vi "Wait For Command.vi"(8 "error in (no error)":errorcluster, 9 "timeout in ms (0)":i32, 11 "Interface in":refnum<class "Interface.lvclass">) -> (0 "error out":errorcluster, 1 "timed out?":bool, 2 "command":T1, 3 "Interface out":refnum<class "Interface.lvclass">, 4 "# elements":u32)   [LabVIEW 2017, in "DSF Core.lvlib" / "Interface.lvclass"]
uses:
  Interface.lvclass
  RT FIFO Data.ctl
  RT FIFO Parameters.ctl
  Interface.lvclass/Interface.ctl
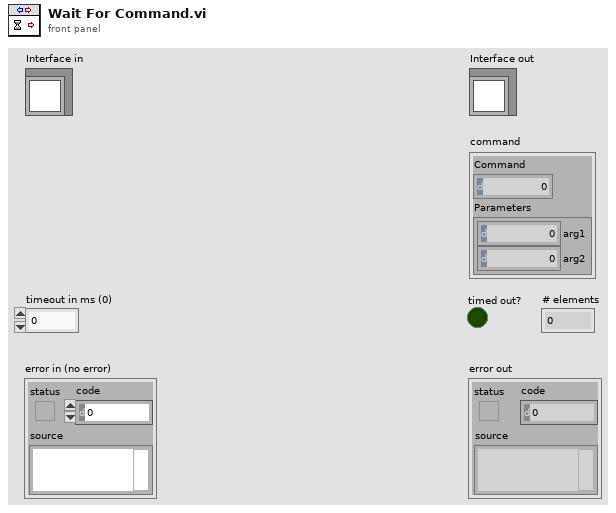
[diagram p1: front panel]
types:
  T1 = typedef "DSF Core.lvlib/Interface.lvclass/RT FIFO Data.ctl" = cluster{"Command":u8, "Parameters":T2}
  T2 = typedef "DSF Core.lvlib/Interface.lvclass/RT FIFO Parameters.ctl" = cluster{"arg1":u64, "arg2":u64}
  T3 = typedef "DSF Core.lvlib/DSF FIFO Options.ctl" = cluster{"Infinite Timeouts":bool}
  T4 = typedef "DSF Core.lvlib/Interface.lvclass/RT FIFO Ref.ctl" = refnum<k33>
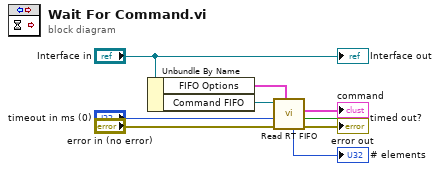
[diagram p0: block diagram]
diagram:
  n1 = Unbundle By Name("Interface in") -> ("FIFO Options"=w1:T3, "Command FIFO"=w2:T4)
  n2 = call "Read RT FIFO.vi"("FIFO Options"=w1, "error in (no error)"="error in (no error)", "timeout in ms (0)"="timeout in ms (0)", "RT FIFO in"=w2) -> ("error out"=→"error out":errorcluster, "empty?"=→"timed out?":bool, "element out"=→"command":T1, "# elements"=→"# elements":u32)  [unwired: 3 in, 1 out]
  "Interface out" <- "Interface in"
